vi "DialogSpeed.vi"(1 "error in (no error)":errorcluster caption="Fehler (Eingang, kein Fehler)", 2 "lLSID":i32) -> (0 "error out":errorcluster caption="Fehler (Ausgang)")   [LabVIEW 2018]
uses:
  <userlib>/TANGO_DLL/Tango_DLL.lvlib
panel:
  in  "Abort":bool
  in  "Set":bool
  in  "Velocity A-Axis":dbl format="%_4g"
  in  "Velocity Z-Axis":dbl format="%_4g"
  in  "Velocity Y-Axis":dbl format="%_4g"
  in  "Acceleration A-Axis":dbl format="%_4g"
  in  "Acceleration Z-Axis":dbl format="%_4g"
  in  "Acceleration Y-Axis":dbl format="%_4g"
  in  "Velocity X-Axis":dbl format="%_4g"
  in  "Acceleration X-Axis":dbl format="%_4g"
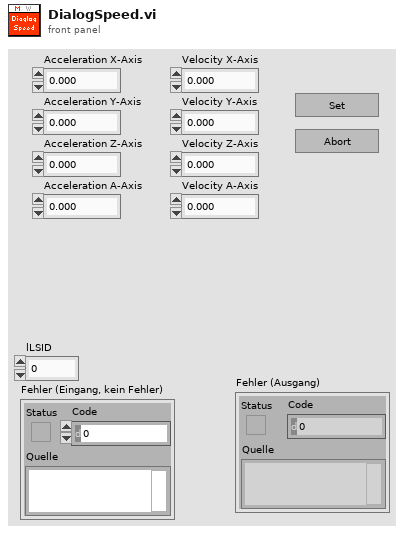
[diagram p1: front panel]
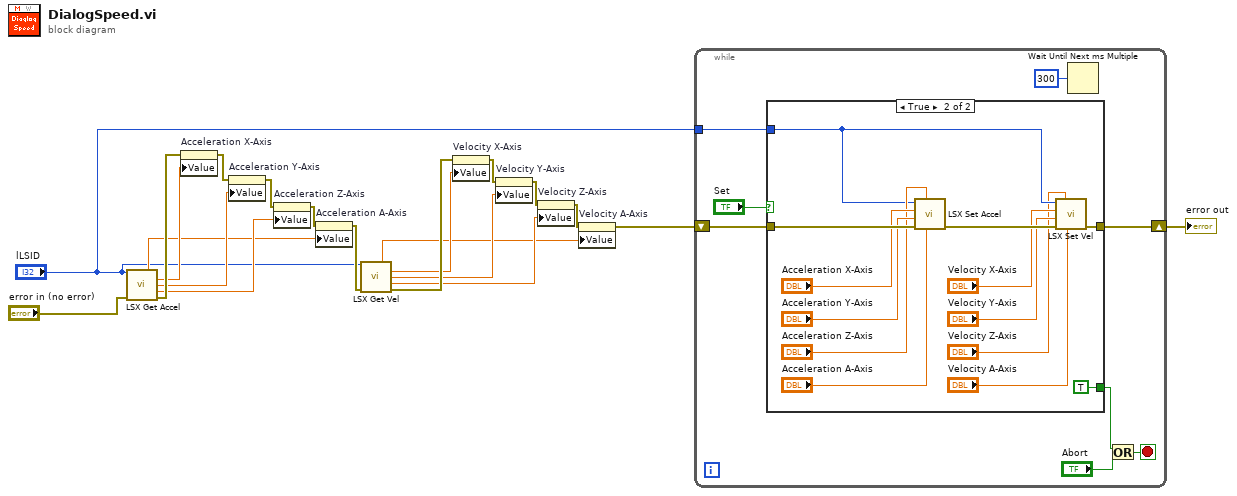
[diagram p0: block diagram]
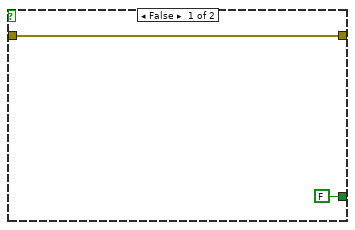
[diagram p2: hidden frame]
diagram:
  n1 = call <userlib>:"LSX Get Accel.vi"("lLSID"="lLSID", "error in (no error)"="error in (no error)") -> ("pdA out"=w13:dbl, "pdX out"=w16:dbl, "pdY out"=w15:dbl, "pdZ out"=w14:dbl, "error out"=w20:errorcluster)  [unwired: 8 in, 1 out]
  n2 = property on="Acceleration X-Axis" class="DigNum (strict)"(error in=w20, "Value"=w16) -> (error out=w19:errorcluster)  [unwired: 1 in, 1 out]
  n3 = property on="Acceleration Y-Axis" class="DigNum (strict)"(error in=w19, "Value"=w15) -> (error out=w18:errorcluster)  [unwired: 1 in, 1 out]
  n4 = property on="Acceleration Z-Axis" class="DigNum (strict)"(error in=w18, "Value"=w14) -> (error out=w17:errorcluster)  [unwired: 1 in, 1 out]
  n5 = property on="Acceleration A-Axis" class="DigNum (strict)"(error in=w17, "Value"=w13) -> (error out=w12:errorcluster)  [unwired: 1 in, 1 out]
  n6 = call <userlib>:"LSX Get Vel.vi"("lLSID"="lLSID", "error in (no error)"=w12) -> ("pdA out"=w4:dbl, "pdX out"=w7:dbl, "pdY out"=w6:dbl, "pdZ out"=w5:dbl, "error out"=w9:errorcluster)  [unwired: 8 in, 1 out]
  n7 = property on="Velocity X-Axis" class="DigNum (strict)"(error in=w9, "Value"=w7) -> (error out=w11:errorcluster)  [unwired: 1 in, 1 out]
  n8 = property on="Velocity Y-Axis" class="DigNum (strict)"(error in=w11, "Value"=w6) -> (error out=w8:errorcluster)  [unwired: 1 in, 1 out]
  n9 = property on="Velocity Z-Axis" class="DigNum (strict)"(error in=w8, "Value"=w5) -> (error out=w10:errorcluster)  [unwired: 1 in, 1 out]
  n10 = property on="Velocity A-Axis" class="DigNum (strict)"(error in=w10, "Value"=w4) -> (error out=w3:errorcluster)  [unwired: 1 in, 1 out]
  n11 = while {
    tunnel: "lLSID" -> [w26]
    shift-right: [w22] -> w1
    shift-left: w3 -> [w27]
    stop <- w24 stop-if-true
    n12 = case shown="True" "Set" {
      tunnel: w27 -> [w31 w44]
      tunnel: w26 -> [_ w38]
      tunnel: [FALSE TRUE] -> w25
      tunnel: [w31 w32] -> w22
      frame False {
      }
      frame True {
        n13 = call <userlib>:"LSX Set Accel.vi"("dA"="Acceleration A-Axis", "dZ"="Acceleration Z-Axis", "error in (no error)"=w44, "dY"="Acceleration Y-Axis", "dX"="Acceleration X-Axis", "lLSID"=w38) -> ("error out"=w39:errorcluster)  [unwired: 4 in, 1 out]
        n14 = call <userlib>:"LSX Set Vel.vi"("dA"="Velocity A-Axis", "dZ"="Velocity Z-Axis", "error in (no error)"=w39, "dY"="Velocity Y-Axis", "dX"="Velocity X-Axis", "lLSID"=w38) -> ("error out"=w32:errorcluster)  [unwired: 4 in, 1 out]
      }
    }
    n15 = Wait Until Next ms Multiple(millisecond multiple=u32 300 ("Vielfache von ms")) -> ()  [unwired: 1 out]
    n16 = Or(x=w25, y="Abort") -> (x .or. y?=w24:bool)
  }
  "error out" <- w1
